vi "User Access Level FGV.vi"(7 "Enum":T1, 8 "Error In":errorcluster, 10 "User Name":string) -> (0 "Error Out":errorcluster, 1 "User Level":string)   [LabVIEW 2018]
doc: "This FGV holds the Access Level for the user currently logged in. It executes the following methods:\n\n1. <B>Read User Access Level File:</B> Reads a tab-delimited text file containing User Names and corresponding Access Levels.\n2. <B>Set Current Access Level:</B> Sets the Access level for the User Name input.\n3. <B>Get Current Access Level:</B> Returns the Access level for the current User."
uses:
  Solutions/Exercise 3-2/User Level FGV/User Level Cmd.ctl
  <vilib>/Utility/file.llb/Read Delimited Spreadsheet (string).vi
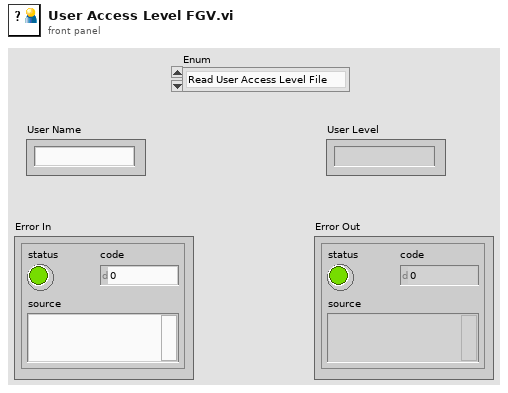
[diagram p1: front panel]
types:
  T1 = typedef "User Level Cmd.ctl" = enum16{"Read User Access Level File", "Set Current User", "Get User Access Level"}
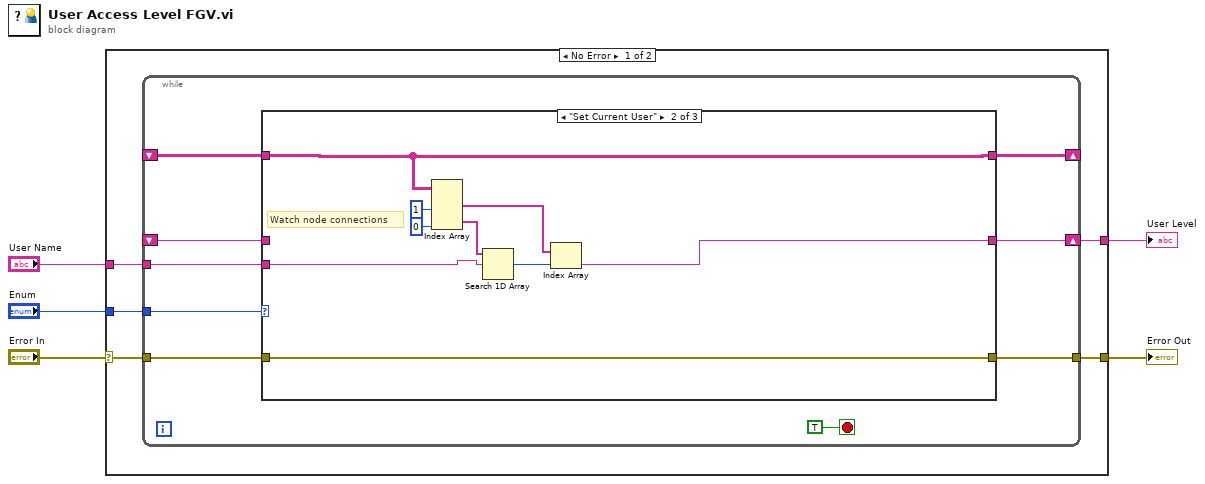
[diagram p0: block diagram]
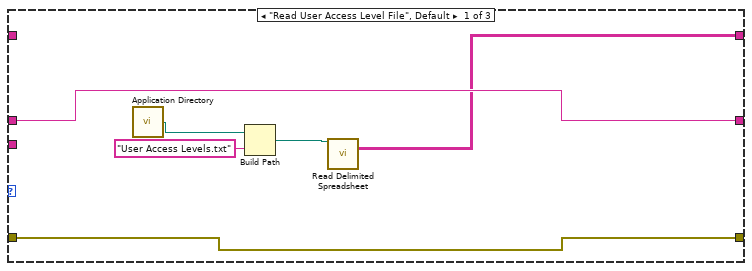
[diagram p2: hidden frame]
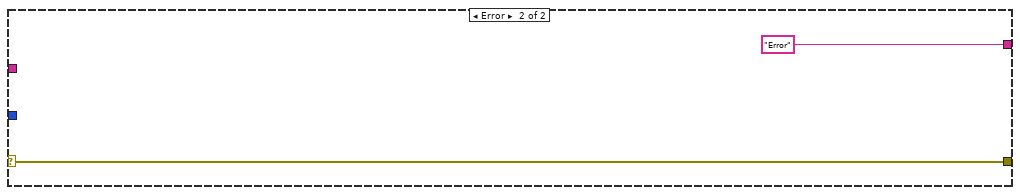
[diagram p4: hidden frame]
diagram:
  n1 = case shown="No Error" "Error In" {
    selector: "Error In" -> [w10 w38]
    tunnel: [w9 w38] -> w4
    tunnel: "Enum" -> [w8 _]
    tunnel: "User Name" -> [w7 _]
    tunnel: [w6 "Error" ("String")] -> w1
    frame No Error {
      n2 = while {
        tunnel: w10 -> [w19]
        tunnel: [w18] -> w9
        tunnel: w8 -> [w17]
        shift-right: [w15] -> _
        shift-left: _ -> [w14]
        tunnel: w7 -> [w13]
        shift-right: [w12] -> w6
        shift-left: _ -> [w11]
        stop <- TRUE stop-if-true
        n3 = case shown="\"Set Current User\"" w17 {
          tunnel: w19 -> [w23 w34 w37]
          tunnel: [w23 w34 w37] -> w18
          tunnel: [w21 w26 w36] -> w15
          tunnel: w14 -> [_ w26 w36]
          tunnel: w13 -> [_ w29 _]
          tunnel: [w22 w32 w35] -> w12
          tunnel: w11 -> [w22 _ w35]
          frame "Read User Access Level File", Default {
            n4 = call <vilib>:"Application Directory.vi"() -> ("Application Directory"=w20:path)
            n5 = Build Path(base path=w20, name or relative path="User Access Levels.txt") -> (appended path=w24:path)
            n6 = call-poly <vilib>:"Read Delimited Spreadsheet.vi"("file path (dialog if empty)"=w24) -> ("all rows"=w21:string[][])  [unwired: 9 in, 5 out]
          }
          frame "Set Current User" {
            # "Watch node connections"
            n7 = Index Array(array=w26, index (col) #1=1 ("disabled index (col)"), index (col) #2=0 ("index (col)")) -> (element #1=w31:string[], element #2=w30:string[])  [unwired: 2 in]
            n8 = Search 1D Array(1D array=w30, element=w29) -> (index of element=w33:i32)  [unwired: 1 in]
            n9 = Index Array(array=w31, index=w33) -> (element=w32:string)
          }
          frame "Get User Access Level" {
          }
        }
      }
    }
    frame Error {
    }
  }
  "User Level" <- w1
  "Error Out" <- w4
